vi "setHashFunction.vi"(8 "error in (no error)":errorcluster, 10 "Hash Function":refnum<vi>, 11 "HashMap in":refnum<class "HashMap.lvclass">) -> (0 "error out":errorcluster, 3 "HashMap out":refnum<class "HashMap.lvclass">)   [LabVIEW 2017, in "HashMap.lvclass"]
uses:
  <userlib>/836-Library/Data_Structures/HashMap/HashMap.lvclass
  <userlib>/836-Library/Data_Structures/HashMap/HashMap.lvclass/HashMap.ctl
  <vilib>/Utility/error.llb/Error Cluster From Error Code.vi
  <vilib>/ErrorRing/Error Ring.xnode
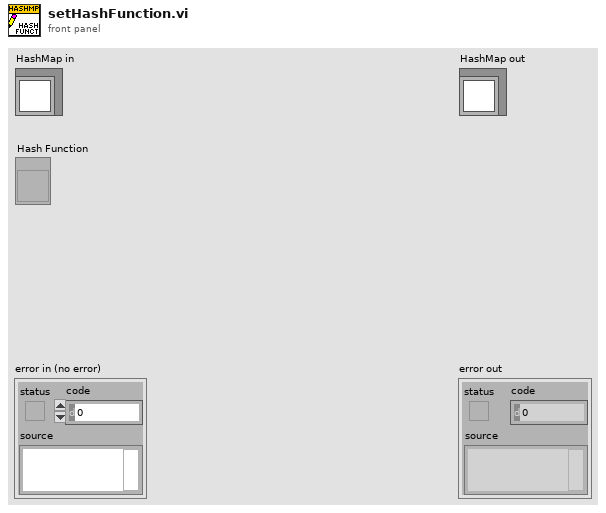
[diagram p1: front panel]
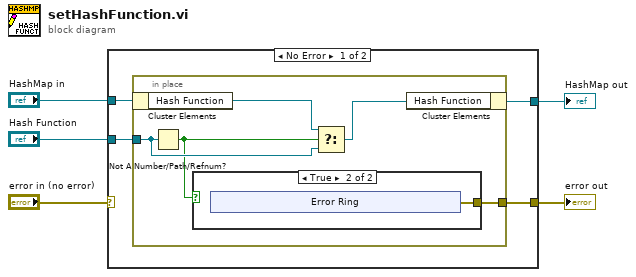
[diagram p0: block diagram]
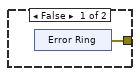
[diagram p2: hidden frame]
diagram:
  n1 = case shown="No Error" "error in (no error)" {
    selector: "error in (no error)" -> [_ w23]
    tunnel: [w6 w23] -> w4
    tunnel: [w8 w24] -> w2
    tunnel: "HashMap in" -> [w9 w24]
    tunnel: "Hash Function" -> [w7 _]
    frame No Error {
      n2 = in-place {
        in-place-border: w7 -> [w12]
        in-place-border: [w10] -> w6
        n3 = in-place-cluster #1(w9) -> ("Hash Function"=w14:refnum<vi>)
        n4 = Not A Number/Path/Refnum?(number/path/refnum=w12) -> (NaN/Path/Refnum?=w11:bool)
        n5 = case shown="True" w11 {
          tunnel: [w15 w17] -> w10
          frame False {
            n6 = xnode "Error Ring"() -> ("error out"=w15:errorcluster)
          }
          frame True {
            n7 = xnode "Error Ring"() -> ("error out"=w17:errorcluster)
          }
        }
        n8 = Select(t=w14, s=w11, f=w12) -> (s? t:f=w13:refnum<vi>)
        n9 = in-place-cluster #1("Hash Function"=w13) -> (w8:refnum<class "HashMap.lvclass">)
      }
    }
    frame Error {
    }
  }
  "error out" <- w4
  "HashMap out" <- w2
